vi "GOOP_ReadClassSettingsFromFile.vi"(8 "error in (no error)":errorcluster, 11 "LvClassPath":path) -> (0 "error out":errorcluster, 2 "ItemIcon":string, 3 "LvClassIconSettings":T1 {"Frame thickness" min=1 max=3 step=1})   [LabVIEW 2016]
uses:
  <resource>/Framework/Providers/Open_GDS/ClassProviders/Common/LvClass_class/GDSLvClass_IconSettingsType.ctl
  <resource>/Framework/Providers/Open_GDS/ClassProviders/Common/LvClass_class/GDSLvClass_IconSettingsNames.ctl
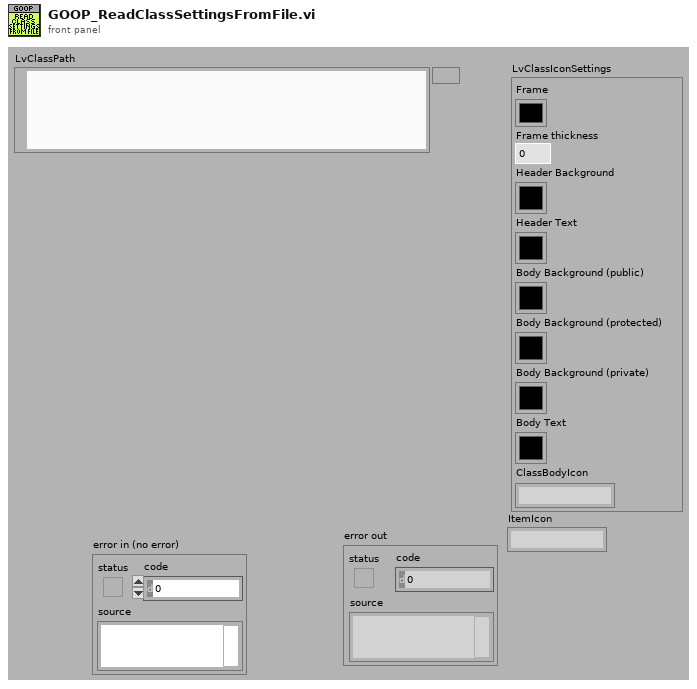
[diagram p1: front panel]
types:
  T1 = typedef "GDSLvClass_IconSettingsType.ctl" = cluster{"Frame":u32, "Frame thickness":u8, "Header Background":u32, "Header Text":u32, "ColorPublic":u32, "ColorProtected":u32, "ColorPrivate":u32, "Body Text":u32, "ClassBodyIcon":string}
  T2 = typedef "GDSLvClass_IconSettingsNames.ctl" = enum16{"EndevoGOOP_ColorFrame", "EndevoGOOP_FrameThickness", "EndevoGOOP_ColorHeader", "EndevoGOOP_ColorTextHeader", "EndevoGOOP_ColorPublic", "EndevoGOOP_ColorProtected", "EndevoGOOP_ColorPrivate", "EndevoGOOP_ColorTextBody", "EndevoGOOP_ClassItemIcon", "EndevoGOOP_ClassBodyIcon"}
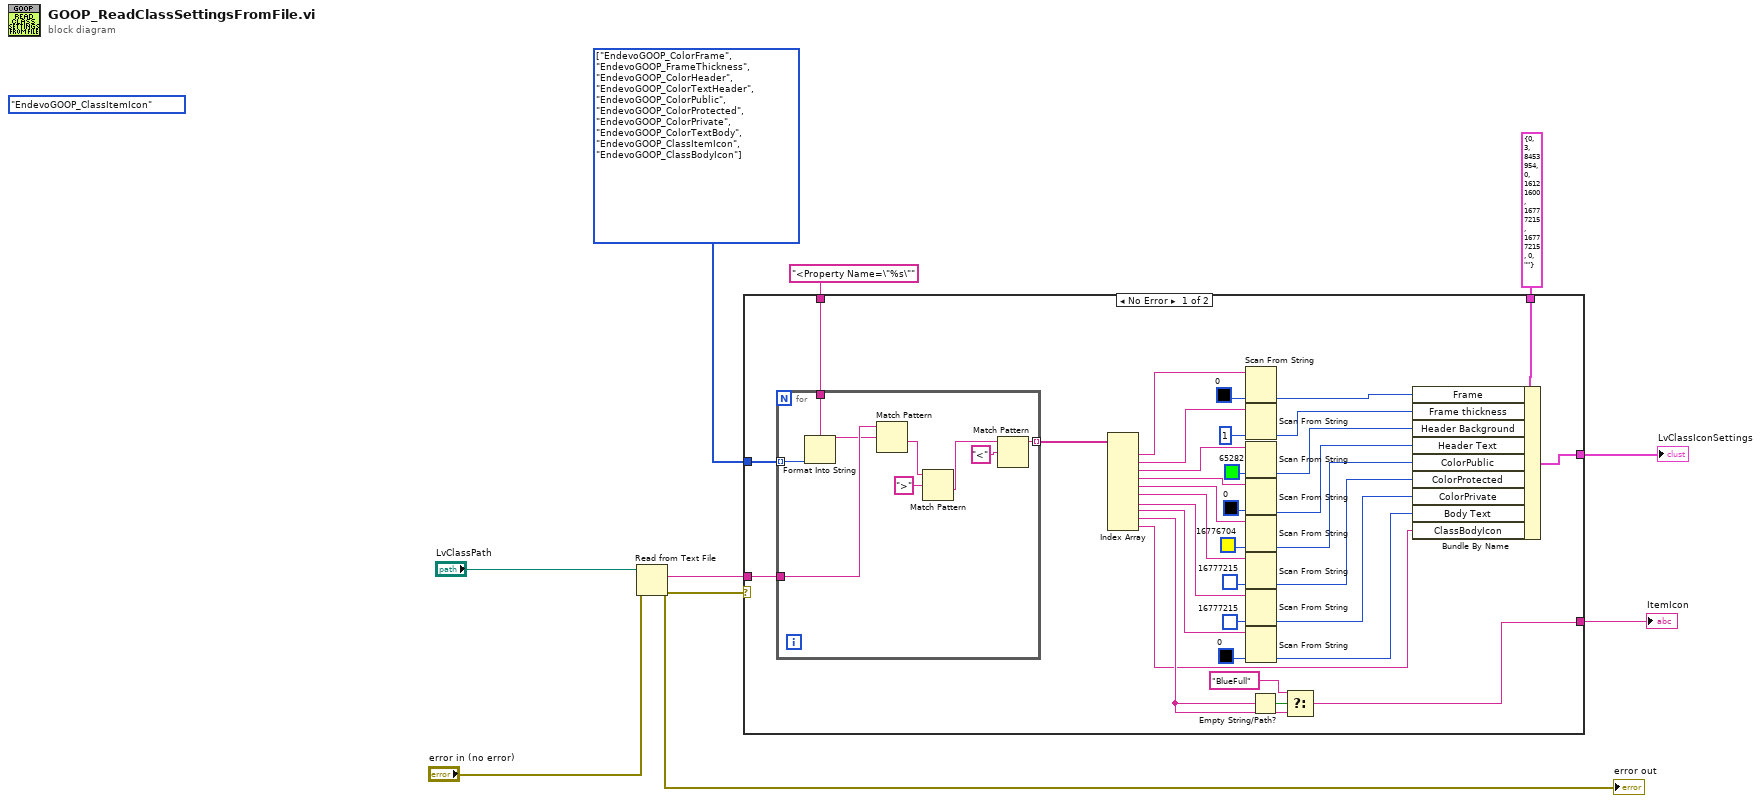
[diagram p0: block diagram]
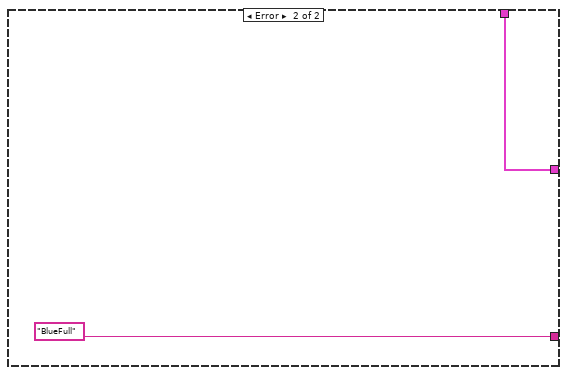
[diagram p2: hidden frame]
diagram:
  w9 = T2[] [enum."EndevoGOOP_ColorFrame", enum."EndevoGOOP_FrameThickness", enum."EndevoGOOP_ColorHeader", enum."EndevoGOOP_ColorTextHeader", enum."EndevoGOOP_ColorPublic", enum."EndevoGOOP_ColorProtected", enum."EndevoGOOP_ColorPrivate", enum."EndevoGOOP_ColorTextBody", enum."EndevoGOOP_ClassItemIcon", enum."EndevoGOOP_ClassBodyIcon"] items=["EndevoGOOP_ColorFrame", "EndevoGOOP_FrameThickness", "EndevoGOOP_ColorHeader", "EndevoGOOP_ColorTextHeader", "EndevoGOOP_ColorPublic", "EndevoGOOP_ColorProtected", "EndevoGOOP_ColorPrivate", "EndevoGOOP_ColorTextBody", "EndevoGOOP_ClassItemIcon", "EndevoGOOP_ClassBodyIcon"]
  (unwired) GDSLvClass_IconSettingsNames."EndevoGOOP_ClassItemIcon" ("Enum")
  n1 = Read from Text File(file (use dialog)="LvClassPath", error in="error in (no error)") -> (text=w7:string, error out=w2:errorcluster)  [unwired: 2 in, 2 out]
  "error out" <- w2
  n2 = case shown="No Error" w2 {
    tunnel: w9 -> [w44 _]
    tunnel: "<Property Name=\"%s\"" ("format string") -> [w43 _]
    tunnel: w7 -> [w42 _]
    tunnel: [w40 w54] -> w5
    tunnel: [w18 "BlueFull"] -> w4
    tunnel: T1 {"Frame"=0, "Frame thickness"=3, "Header Background"=8453954, "Header Text"=0, "ColorPublic"=16121600, "ColorProtected"=16777215, "ColorPrivate"=16777215, "Body Text"=0, "ClassBodyIcon"=""} ("LvClassIconSettings") -> [w41 w54]
    frame No Error {
      n3 = for {
        tunnel: w44 -> [w53] mode=indexing
        tunnel: w43 -> [w52]
        tunnel: w42 -> [w51]
        tunnel: [w48] -> w39 mode=indexing
        n4 = Format Into String(format string=w52, w53) -> (resulting string=w50:string)  [unwired: 2 in, 1 out]
        n5 = Match Pattern(string=w51, regular expression=w50) -> (after substring=w46:string)  [unwired: 1 in, 3 out]
        n6 = Match Pattern(string=w46, regular expression=">") -> (after substring=w45:string)  [unwired: 1 in, 3 out]
        n7 = Match Pattern(string=w45, regular expression="<") -> (before substring=w48:string)  [unwired: 1 in, 3 out]
      }
      n8 = Index Array(array=w39) -> (element #1=w38:string, element #2=w34:string, element #3=w33:string, element #4=w32:string, element #5=w31:string, element #6=w30:string, element #7=w29:string, element #8=w28:string, element #9=w19:string, element #10=w10:string)  [unwired: 10 in]
      n9 = Scan From String(input string=w38, default 1=u32 0 ("Frame")) -> (output 1=w37:u32)  [unwired: 3 in, 3 out]
      n10 = Scan From String(input string=w34, default 1=u8 1 ("Frame thickness")) -> (output 1=w11:u8)  [unwired: 3 in, 3 out]
      n11 = Scan From String(input string=w33, default 1=u32 65282 ("Frame")) -> (output 1=w12:u32)  [unwired: 3 in, 3 out]
      n12 = Scan From String(input string=w32, default 1=u32 0 ("Frame")) -> (output 1=w13:u32)  [unwired: 3 in, 3 out]
      n13 = Scan From String(input string=w31, default 1=u32 16776704 ("Frame")) -> (output 1=w14:u32)  [unwired: 3 in, 3 out]
      n14 = Scan From String(input string=w30, default 1=u32 16777215 ("Frame")) -> (output 1=w15:u32)  [unwired: 3 in, 3 out]
      n15 = Scan From String(input string=w29, default 1=u32 16777215 ("Frame")) -> (output 1=w16:u32)  [unwired: 3 in, 3 out]
      n16 = Scan From String(input string=w28, default 1=u32 0 ("Frame")) -> (output 1=w17:u32)  [unwired: 3 in, 3 out]
      n17 = Empty String/Path?(string/path=w19) -> (empty?=w21:bool)
      n18 = Select(t="BlueFull", s=w21, f=w19) -> (s? t:f=w18:string)
      n19 = Bundle By Name(cluster=w41, "Frame"=w37, "Frame thickness"=w11, "Header Background"=w12, "Header Text"=w13, "ColorPublic"=w14, "ColorProtected"=w15, "ColorPrivate"=w16, "Body Text"=w17, "ClassBodyIcon"=w10) -> (w40:T1)
    }
    frame Error {
    }
  }
  "ItemIcon" <- w4
  "LvClassIconSettings" <- w5
